vi "NMR_Short_RF_Pulse_Sequence_V2.vi"() -> ()   [LabVIEW 2020]
uses:
  <instrlib>/niFgen/niFgen.llb/niFgen Output Mode.ctl
  <instrlib>/niFgen/niFgen.llb/niFgen Trigger Mode.ctl
  <instrlib>/niFgen/niFgen.llb/niFgen_ctl Trigger DigEdge - Edge Values (Ring).ctl
  <instrlib>/niFgen/niFgen.llb/niFgen_ctl Trigger Source Values (Ring).ctl
  <instrlib>/niFgen/niFgen.llb/niFgen Configure Digital Edge Start Trigger.vi
  <instrlib>/niFgen/niFgen.llb/niFgen Create Waveform (I16).vi
panel:
  in  "Sample Rate":dbl=50000000.0 format="%.2p"
  in  "Waveform Information Array":T1(array[cluster])=[{"Waveform Type"=7, "Amplitude"=-0.5, "# of points"=100}, {"Waveform Type"=3, "Amplitude"=0.5, "# of points"=600}, {"Waveform Type"=7, "Amplitude"=-0.5, "# of points"=245000}, {"Waveform Type"=3, "Amplitude"=0.5, "# of points"=1200}, {"Waveform Type"=7, "Amplitude"=-0.5, "# of points"=495000}, {"Waveform Type"=3, "Amplitude"=0.5, "# of points"=1200}, {"Waveform Type"=7, "Amplitude"=-0.5, "# of points"=490000}, {"Waveform Type"=3, "Amplitude"=0.5, "# of points"=1200}, {"Waveform Type"=7, "Amplitude"=-0.5, "# of points"=485000}, {"Waveform Type"=3, "Amplitude"=0.5, "# of points"=1200}, {"Waveform Type"=7, "Amplitude"=-0.5, "# of points"=1000000}] {"Amplitude" min=0.0 max=1.0 format="%.2f"; "Waveform Type" items=["Sine", "Cosine", "Triangle", "Square", "Sawtooth", "Increasing Ramp", "Decreasing Ramp", "DC Value"]}
  in  "Gain":dbl(knob)=1.0 min=0.0 max=5.0 scale=0.0..5.0 scale format="%#.1f"
  in  "FGEN Resource Name 2":refnum<k15>="FGEN2" caption="FGEN Resource Name"
  in  "Frequency":dbl=27510000.0 format="%.4p"
  in  "Amplitude":dbl=0.35 format="%0_3g"
  in  "Marker Output Behavior":i32(ring)=101 items=["Pulse"=101, "Toggle"=103]
  in  "Marker Output Terminal":string(combo)="PFI0"
  in  "Waveform Marker Position":i32
  in  "FGEN Resource Name":refnum<k15>="Dev1"
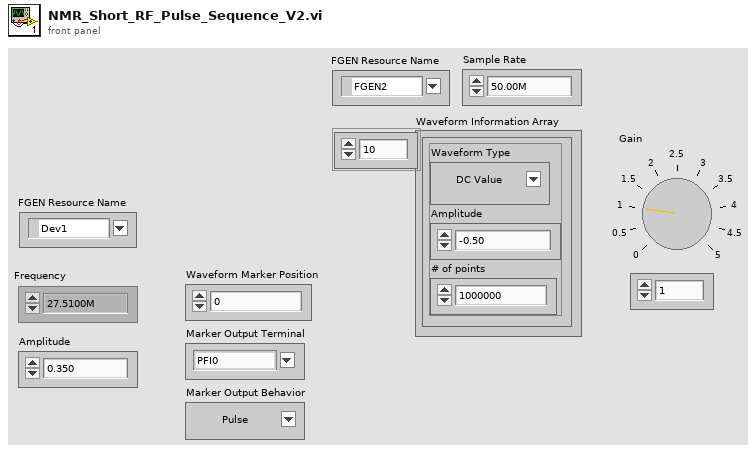
[diagram p1: front panel]
types:
  T1 = cluster{"Waveform Type":u16, "Amplitude":dbl, "# of points":u32}[]
  T2 = typedef "niFgen_ctl Trigger Source Values (Ring).ctl" = string
  T3 = typedef "niFgen_ctl Trigger DigEdge - Edge Values (Ring).ctl" = i32
  T4 = typedef "niFgen Trigger Mode.ctl" = i32
  T5 = typedef "niFgen Output Mode.ctl" = u32
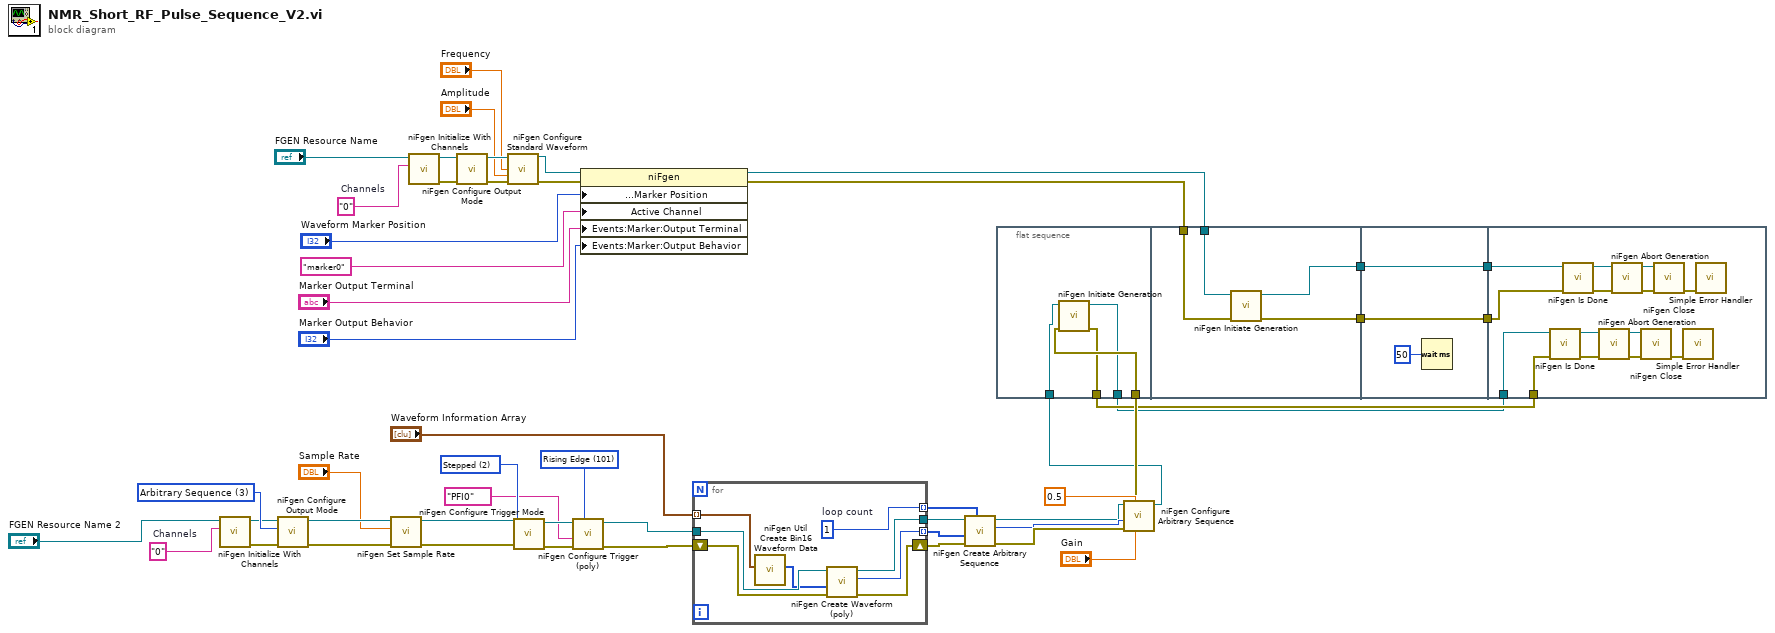
[diagram p0: block diagram]
diagram:
  w18 = T3 101 items=["Rising Edge"=101, "Falling Edge"=102] ("Edge (Rising)")
  w19 = T4 2 items=["Single", "Continuous", "Stepped", "Burst"] ("Trigger Mode (default: 1=continuous)")
  w25 = "0"  # Channels
  w31 = T5 3 items=["Standard Function", "Frequency List", "Arbitrary Waveform", "Arbitrary Sequence", "Script"] ("output mode")
  w44 = "0"  # Channels
  n1 = call <instrlib>:"niFgen Initialize With Channels.vi"("Channel Name"=w25, "Resource Name"="FGEN Resource Name 2") -> ("error out"=w28:errorcluster, "Instrument Handle Out"=w27:refnum<k15>)  [unwired: 8 in]
  n2 = call <instrlib>:"niFgen Configure Output Mode.vi"("error in (no error)"=w28, "Output Mode (default: 0=Standard Function)"=w31, "Instrument Handle"=w27) -> ("error out"=w14:errorcluster, "Instrument Handle Out"=w15:refnum<k15>)  [unwired: 6 in]
  n3 = call <instrlib>:"niFgen Set Sample Rate.vi"("error in (no error)"=w14, "Sample Rate (Samp/s)"="Sample Rate", "Instrument Handle"=w15) -> ("error out"=w12:errorcluster, "Instrument Handle Out"=w13:refnum<k15>)  [unwired: 7 in]
  n4 = call <instrlib>:"niFgen Initialize With Channels.vi"("Channel Name"=w44, "Resource Name"="FGEN Resource Name") -> ("error out"=w46:errorcluster, "Instrument Handle Out"=w47:refnum<k15>)  [unwired: 8 in]
  n5 = call <instrlib>:"niFgen Configure Output Mode.vi"("error in (no error)"=w46, "Instrument Handle"=w47) -> ("error out"=w42:errorcluster, "Instrument Handle Out"=w43:refnum<k15>)  [unwired: 7 in]
  n6 = call <instrlib>:"niFgen Configure Standard Waveform.vi"("Instrument Handle"=w43, "Frequency"="Frequency", "Amplitude"="Amplitude", "error in (no error)"=w42) -> ("Instrument Handle Out"=w39:refnum<k15>, "error out"=w38:errorcluster)  [unwired: 10 in]
  n7 = call <instrlib>:"niFgen Configure Trigger Mode.vi"("error in (no error)"=w12, "Trigger Mode (default: 1=continuous)"=w19, "Instrument Handle"=w13) -> ("error out"=w22:errorcluster, "Instrument Handle Out"=w23:refnum<k15>)  [unwired: 7 in]
  n8 = call-poly <instrlib>:"niFgen Configure Trigger (poly).vi"("Edge (Rising)"=w18, "error in (no error)"=w22, "Source"=T2 "PFI0", "Instrument Handle"=w23) -> ("error out"=w20:errorcluster, "Instrument Handle Out"=w21:refnum<k15>)  [unwired: 6 in]
  n9 = property class="niFgen"(reference=w39, error in=w38, "Arbitrary Waveform:Arbitrary Waveform Mode:Marker Position"="Waveform Marker Position", "Active Channel"="marker0", "Events:Marker:Output Terminal"="Marker Output Terminal", "Events:Marker:Output Behavior"="Marker Output Behavior") -> (reference out=w10:refnum<k15>, error out=w11:errorcluster)
  n10 = for {
    shift-right: [w58] -> w32
    shift-left: w20 -> [w56]
    tunnel: [w59] -> w33
    tunnel: w21 -> [w57]
    tunnel: [w55] -> w34 mode=indexing
    tunnel: "Waveform Information Array" -> [w53] mode=indexing
    tunnel: [w52] -> w30 mode=indexing
    w52 = 1  # loop count
    n11 = call <instrlib>:"niFgen Util Create Bin16 Waveform Data.vi"("Waveform"=w53) -> ("Waveform Data"=w54:i16[])  [unwired: 10 in]
    n12 = call-poly <instrlib>:"niFgen Create Waveform (poly).vi"("error in (no error)"=w56, "Waveform Data Array"=w54, "Instrument Handle"=w57) -> ("error out"=w58:errorcluster, "Waveform Handle"=w55:i32, "Instrument Handle Out"=w59:refnum<k15>)  [unwired: 6 in]
  }
  n13 = call <instrlib>:"niFgen Create Arbitrary Sequence.vi"("Loop Counts Array"=w30, "error in (no error)"=w32, "Waveform Handles Array"=w34, "Instrument Handle"=w33) -> ("error out"=w37:errorcluster, "Sequence Handle"=w36:i32, "Instrument Handle Out"=w35:refnum<k15>)  [unwired: 5 in]
  n14 = flat-sequence {
    tunnel: w9 -> [w63]
    tunnel: w8 -> [w62]
    tunnel: [w61] -> w7
    tunnel: [w60] -> w6
    tunnel: w11 -> [w67]
    tunnel: w10 -> [w66]
    tunnel: [w65] -> w5
    tunnel: [w64] -> w3
    tunnel: w5 -> [w70]
    tunnel: [w70] -> w4
    tunnel: w3 -> [w69]
    tunnel: [w69] -> w2
    tunnel: w4 -> [w82]
    tunnel: w2 -> [w81]
    tunnel: w7 -> [w74]
    tunnel: w6 -> [w73]
    frame #0 {
      n15 = call <instrlib>:"niFgen Initiate Generation.vi"("error in (no error)"=w63, "Instrument Handle"=w62) -> ("error out"=w61:errorcluster, "Instrument Handle Out"=w60:refnum<k15>)  [unwired: 8 in]
    }
    frame #1 {
      n16 = call <instrlib>:"niFgen Initiate Generation.vi"("error in (no error)"=w67, "Instrument Handle"=w66) -> ("error out"=w65:errorcluster, "Instrument Handle Out"=w64:refnum<k15>)  [unwired: 8 in]
    }
    frame #2 {
      n17 = Wait (ms)(milliseconds to wait=u32 50 ("millisecond multiple")) -> ()  [unwired: 1 out]
    }
    frame #3 {
      n18 = call <instrlib>:"niFgen Is Done.vi"("error in (no error)"=w74, "Instrument Handle"=w73) -> ("error out"=w77:errorcluster, "Instrument Handle Out"=w72:refnum<k15>)  [unwired: 7 in, 1 out]
      n19 = call <instrlib>:"niFgen Is Done.vi"("error in (no error)"=w82, "Instrument Handle"=w81) -> ("error out"=w80:errorcluster, "Instrument Handle Out"=w84:refnum<k15>)  [unwired: 7 in, 1 out]
      n20 = call <instrlib>:"niFgen Abort Generation.vi"("error in (no error)"=w77, "Instrument Handle"=w72) -> ("error out"=w76:errorcluster, "Instrument Handle Out"=w71:refnum<k15>)  [unwired: 8 in]
      n21 = call <instrlib>:"niFgen Abort Generation.vi"("error in (no error)"=w80, "Instrument Handle"=w84) -> ("error out"=w79:errorcluster, "Instrument Handle Out"=w83:refnum<k15>)  [unwired: 8 in]
      n22 = call <instrlib>:"niFgen Close.vi"("error in (no error)"=w76, "Instrument Handle"=w71) -> ("error out"=w75:errorcluster)  [unwired: 9 in]
      n23 = call <instrlib>:"niFgen Close.vi"("error in (no error)"=w79, "Instrument Handle"=w83) -> ("error out"=w78:errorcluster)  [unwired: 9 in]
      n24 = call <vilib>:"Simple Error Handler.vi"("error in (no error)"=w75) -> ()  [unwired: 4 in, 5 out]
      n25 = call <vilib>:"Simple Error Handler.vi"("error in (no error)"=w78) -> ()  [unwired: 4 in, 5 out]
    }
  }
  n26 = call <instrlib>:"niFgen Configure Arbitrary Sequence.vi"("Gain"="Gain", "Offset"=0.5, "error in (no error)"=w37, "Sequence Handle"=w36, "Instrument Handle"=w35) -> ("error out"=w9:errorcluster, "Instrument Handle Out"=w8:refnum<k15>)  [unwired: 5 in]
